vi "rawpower2totalprad.vi"(3 "PowerArray [W]":sgl[][](array[numeric]), 4 "No. of Samples\n[TOA / Sample Rate]":u32=10000, 5 "kbolott_and_volume":dbl[][](array[numeric])) -> (0 "full P_rad [MW] HBC":dbl[](array[numeric]), 1 "full P_rad [MW] VBC":dbl[](array[numeric]), 2 "corrected PowerArray":dbl[][](array[numeric]))   [LabVIEW 2014]
panel:
  out "sample2":i32
  out "sample":i32
  out "channel VBC":i32
  out "V_Cam 2":dbl format="%#_13g"
  out "channelListVBC":i32[](array[numeric])
  out "sample array [MW] 2":dbl[](array[numeric])
  out "constant 2":dbl
  out "element 2":sgl
  out "volume/kbolott 2":dbl
  out "element after 2":dbl
  out "kbolott 2":dbl
  out "volume 2":dbl
  out "constant*geom 2":dbl
  out "test plot":cluster{cluster{i32, "element":dbl}[]}[](graph)
  out "Nsample array":i32[](array[numeric])
  out "channel subarray":sgl[](array[numeric])
  out "offset channel":sgl
  out "channel":i32
  out "power size":i32[](array[numeric])
  out "offset size":i32[](array[numeric])
  out "power offset all 128":dbl[](array[numeric])
  out "start subarray":sgl[][](array[numeric])
  in  "channel\noffset":i32
  out "constant*geom":dbl
  out "volume":dbl
  out "kbolott":dbl
  out "element after":dbl
  out "volume/kbolott":dbl
  out "element":sgl
  in  "Nchannels":i32=32
  out "sample array [MW]":dbl[](array[numeric])
  out "constant":dbl
  out "V_Cam":dbl format="%#_13g"
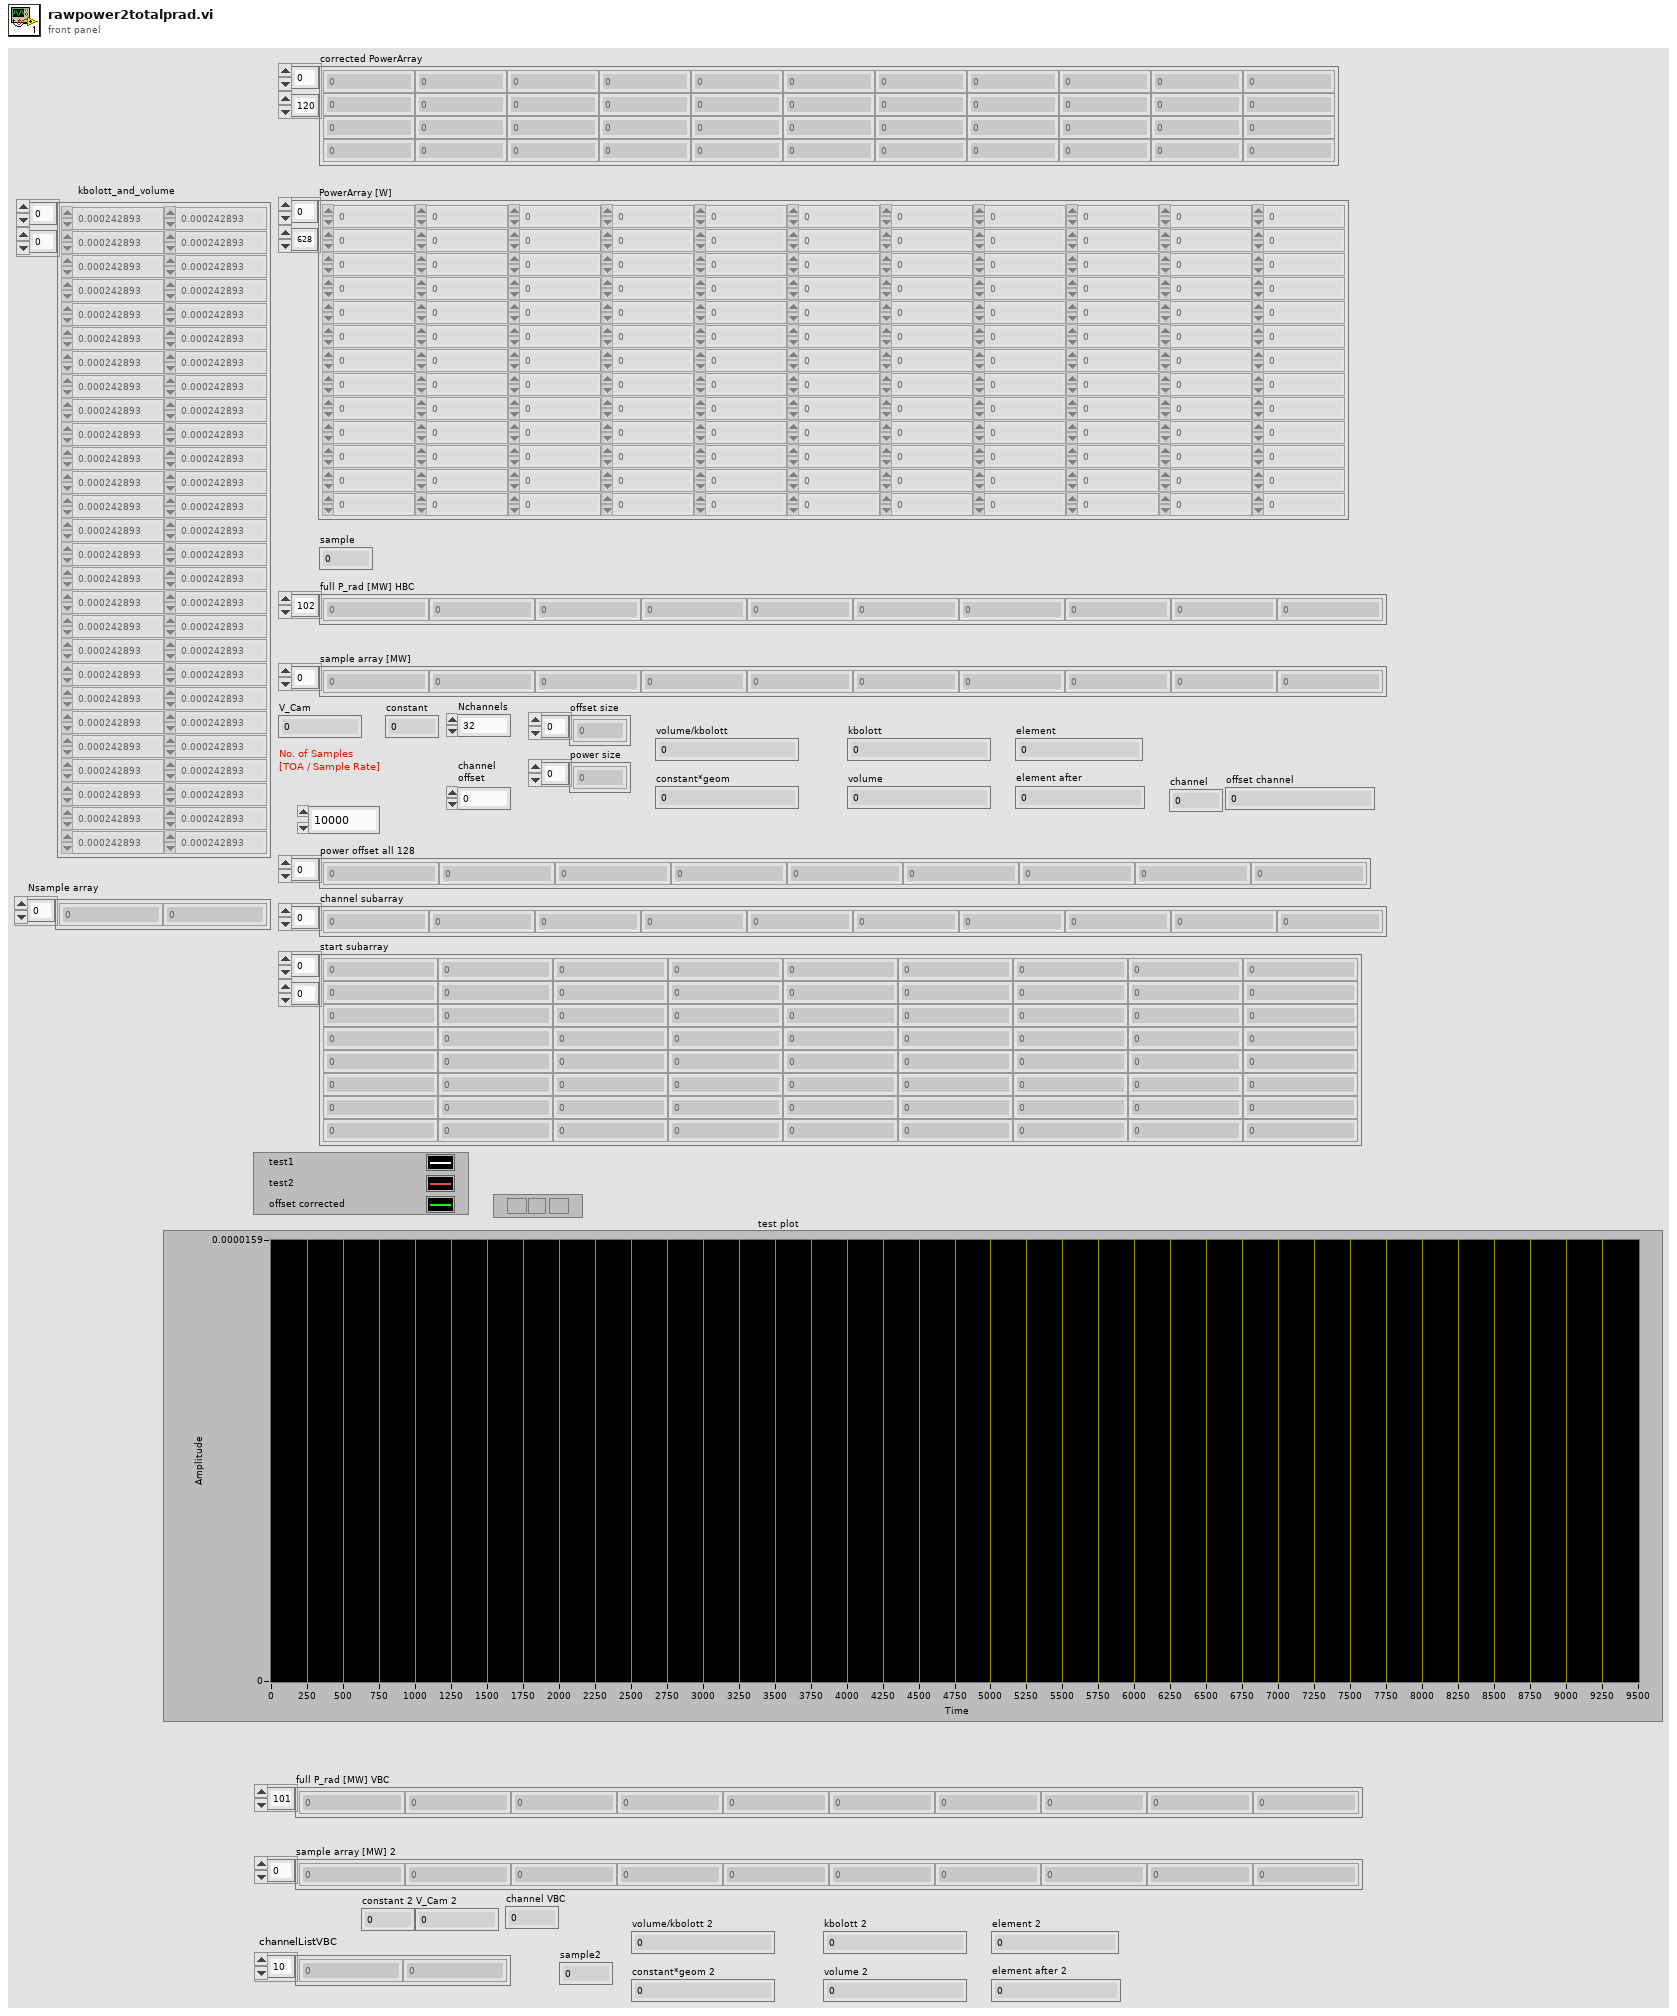
[diagram p1: front panel]
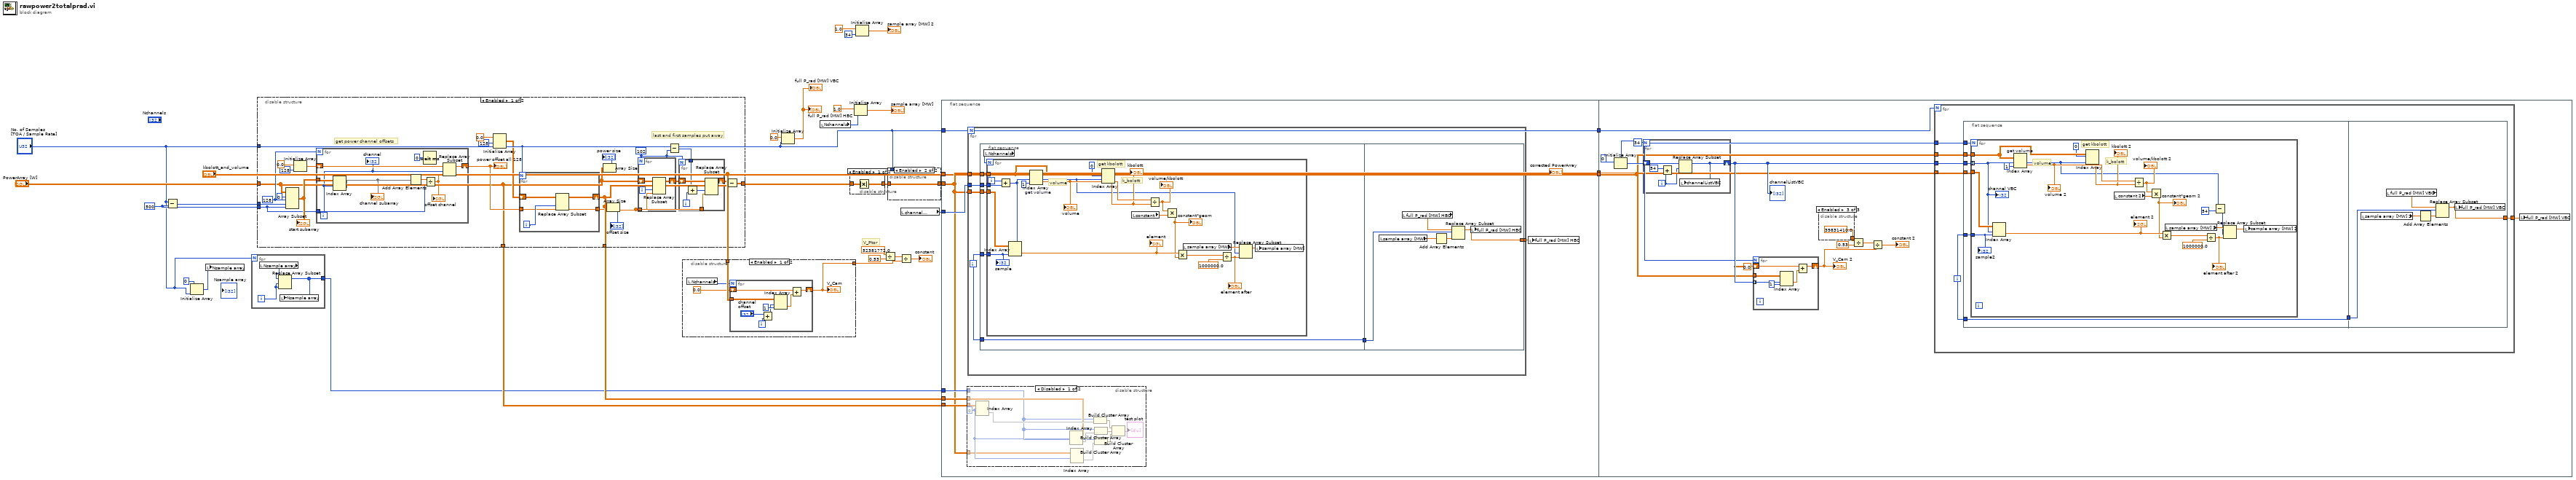
[diagram p0: block diagram]
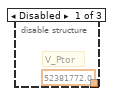
[diagram p3: hidden frame]
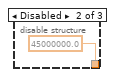
[diagram p4: hidden frame]
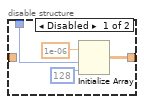
[diagram p7: hidden frame]
diagram:
  w14 = u32 500 ("y")
  # "V_Ptor"
  n1 = Subtract(x="No. of Samples\n[TOA / Sample Rate]", y=w14) -> (x-y=w15:u32)
  n2 = Initialize Array(0, "No. of Samples\n[TOA / Sample Rate]") -> (w19:i32[])
  n3 = local write "Nsample array"(w19) -> ()
  n4 = for {
    N: "No. of Samples\n[TOA / Sample Rate]" -> [_]
    tunnel: [w31] -> w16
    i -> [w32]
    n5 = local read "Nsample array"() -> (w33:i32[])
    n6 = Replace Array Subset(array=w33, new element=w32, index=w32) -> (w31:i32[])
    n7 = local write "Nsample array"(w31) -> ()
  }
  n8 = disable-structure shown="Enabled" {
    disable-tunnel: "PowerArray [W]" -> [w40 w80]
    disable-tunnel: [w43 w80] -> w12
    disable-tunnel: "No. of Samples\n[TOA / Sample Rate]" -> [w36 _]
    disable-tunnel: [w40 _] -> w18
    disable-tunnel: [w44 _] -> w17
    disable-tunnel: w15 -> [w42 _]
    disable-tunnel: w14 -> [w41 _]
    frame Enabled {
      w35 = 102
      w45 = 128 ("length")
      # "last and first samples put away"
      # "get power channel offsets"
      n9 = Array Subset(array=w40, index (row)=0 ("index"), length (row)=w45, index (col)=w42, length (col)=w41) -> (w53:sgl[][])
      "start subarray" <- w53
      n10 = Initialize Array(0.0 ("element"), 128 ("dimension size")) -> (w52:dbl[])
      n11 = for {
        N: w45 -> [_]
        tunnel: w53 -> [w73]
        tunnel: w41 -> [w75]
        shift-right: [w76] -> w49
        shift-left: w52 -> [w78]
        i -> [w72]
        n12 = Index Array(array=w73, index (row)=w72) -> (element=w71:sgl[])  [unwired: 1 in]
        "channel subarray" <- w71
        n13 = Add Array Elements(numeric array=w71) -> (sum=w79:sgl)
        n14 = Wait (ms)(milliseconds to wait=u32 0) -> ()  [unwired: 1 out]
        n15 = Divide(x=w79, y=w75) -> (x/y=w77:sgl)
        "offset channel" <- w77
        n16 = Replace Array Subset(array=w78, new element=w77, index=w72) -> (w76:dbl[])
        "channel" <- w72
      }
      "power offset all 128" <- w49
      n17 = Initialize Array(0.0 ("element"), 128 ("dimension size"), w36) -> (w50:dbl[][])
      n18 = for {
        N: w36 -> [_]
        shift-right: [w68] -> w44
        shift-left: w50 -> [w70]
        tunnel: w49 -> [w67]
        tunnel: [w67] -> w37
        i -> [w69]
        n19 = Replace Array Subset(array=w70, new element=w67, index (col)=w69) -> (w68:dbl[][])  [unwired: 1 in]
      }
      n20 = Array Size(array=w40) -> (size(s)=→"power size":i32[])
      n21 = Array Size(array=w44) -> (size(s)=→"offset size":i32[])
      n22 = for {
        N: w35 -> [_]
        shift-right: [w65] -> w39
        shift-left: w40 -> [w66]
        tunnel: w37 -> [w63]
        i -> [w64]
        n23 = Replace Array Subset(array=w66, new element=w63, index (col)=w64) -> (w65:sgl[][])  [unwired: 1 in]
      }
      n24 = Subtract(x=w36, y=w35) -> (x-y=w34:u32)
      n25 = for {
        N: w35 -> [_]
        shift-right: [w61] -> w38
        shift-left: w39 -> [w62]
        tunnel: w37 -> [w60]
        tunnel: w34 -> [w59]
        i -> [w58]
        n26 = Add(x=w59, y=w58) -> (x+y=w57:u32)
        n27 = Replace Array Subset(array=w62, new element=w60, index (col)=w57) -> (w61:sgl[][])  [unwired: 1 in]
      }
      n28 = Subtract(x=w38, y=w44) -> (x-y=w43:dbl[][])
    }
    frame Disabled {
    }
  }
  n29 = disable-structure shown="Enabled" {
    disable-tunnel: "kbolott_and_volume" -> [w84 _]
    disable-tunnel: [w81 _] -> w22
    frame Enabled {
      n30 = local read "Nchannels"() -> (w83:i32)
      n31 = for {
        N: w83 -> [_]
        tunnel: w84 -> [w92]
        shift-right: [w88] -> w81
        shift-left: 0.0 ("V_Cam") -> [w89]
        i -> [w86]
        n32 = Add(x="channel\noffset", y=w86) -> (x+y=w87:i32)
        n33 = Index Array(array=w92, index (row)=w87, index (col)=1 ("disabled index (col)")) -> (element=w91:dbl)
        n34 = Add(x=w89, y=w91) -> (x+y=w88:dbl)
      }
      "V_Cam" <- w81
    }
    frame Disabled {
    }
  }
  n35 = Initialize Array(0.0 ("element"), "No. of Samples\n[TOA / Sample Rate]") -> (→"full P_rad [MW] HBC" →"full P_rad [MW] VBC":dbl[])
  n36 = local read "Nchannels"() -> (w27:i32)
  n37 = disable-structure shown="Enabled" {
    disable-tunnel: [w94 w95] -> w21
    disable-tunnel: w12 -> [w93 w95]
    frame Enabled {
      n38 = Absolute Value(x=w93) -> (abs(x)=w94:dbl[][])
    }
    frame Disabled {
    }
  }
  n39 = Initialize Array(1.0 ("element"), w27) -> (→"sample array [MW]":dbl[])
  n40 = Initialize Array(1.0 ("element"), 34 ("dimension size")) -> (→"sample array [MW] 2":dbl[])
  n41 = Divide(x=52381772.0, y=0.53) -> (x/y=w25:dbl)
  n42 = disable-structure shown="Enabled" {
    disable-tunnel: "No. of Samples\n[TOA / Sample Rate]" -> [w98 _]
    disable-tunnel: [w96 w100] -> w9
    disable-tunnel: w21 -> [_ w100]
    frame Disabled {
      n43 = Initialize Array(1e-06 ("element"), w98, 128 ("dimension size")) -> (w96:dbl[][])
    }
    frame Enabled {
    }
  }
  n44 = Divide(x=w25, y=w22) -> (x/y=→"constant":dbl)
  n45 = local read "channel\noffset"() -> (w23:i32)
  n46 = flat-sequence {
    tunnel: w23 -> [w108]
    tunnel: w18 -> [w106]
    tunnel: w17 -> [w105]
    tunnel: w16 -> [w104]
    tunnel: w9 -> [w102]
    tunnel: [w103] -> w8
    tunnel: "No. of Samples\n[TOA / Sample Rate]" -> [w103]
    tunnel: [w102] -> w6
    tunnel: [w101] -> w5
    tunnel: "kbolott_and_volume" -> [w101]
    tunnel: w8 -> [w159]
    tunnel: w6 -> [w157]
    tunnel: w5 -> [w158]
    frame #0 {
      n47 = disable-structure shown="Disabled" {
        disable-tunnel: w106 -> [w117 _]
        disable-tunnel: w105 -> [w115 _]
        disable-tunnel: w104 -> [w112 _]
        disable-tunnel: w102 -> [w109 _]
        frame Disabled {
          w111 = 0 ("index (row)")
          n48 = Index Array(array=w117, index (row)=w111) -> (element=w116:sgl[])  [unwired: 1 in]
          n49 = Index Array(array=w115, index (row)=w111) -> (element=w114:dbl[])  [unwired: 1 in]
          n50 = Index Array(array=w109, index (row)=w111) -> (element=w110:dbl[])  [unwired: 1 in]
          n51 = Build Cluster Array(w112, w116) -> (w118:cluster{i32, sgl}[])
          n52 = Build Cluster Array(w112, w114) -> (w120:cluster{i32, "element":dbl}[])
          n53 = Build Cluster Array(w112, w110) -> (w113:cluster{i32, dbl}[])
          n54 = Build Cluster Array(w118, w120, w113) -> (→"test plot":cluster{cluster{i32, "element":dbl}[]}[])
        }
        frame Enabled {
        }
      }
      n55 = for {
        N: w103 -> [_]
        tunnel: w102 -> [w126]
        tunnel: w101 -> [w125]
        tunnel: w108 -> [w122]
        tunnel: [w121] -> w107
        i -> [w123]
        n56 = flat-sequence {
          tunnel: w126 -> [w131]
          tunnel: w125 -> [w130]
          tunnel: w123 -> [w129]
          tunnel: [w128] -> w124
          tunnel: w123 -> [w128]
          tunnel: w122 -> [w127]
          tunnel: w124 -> [w155]
          tunnel: [w152] -> w121
          frame #0 {
            n57 = local read "Nchannels"() -> (w132:i32)
            n58 = for {
              N: w132 -> [_]
              tunnel: w131 -> [w148]
              tunnel: w130 -> [w150]
              tunnel: w129 -> [w147]
              tunnel: w127 -> [w133]
              i -> [w135]
              # "get kbolott"
              # "k_bolott"
              # "volume"
              n59 = Add(x=w135, y=w133) -> (x+y=w134:i32)
              n60 = Index Array(array=w148, index (row)=w134, index (col)=w147) -> (element=w144:dbl)
              "element" <- w144
              n61 = Index Array "get volume"(array=w150, index (row)=w134, index (col)=1 ("disabled index (col)")) -> (element=w142:dbl)
              "volume" <- w142
              n62 = Index Array(array=w150, index (row)=w134, index (col)=0 ("disabled index (col)")) -> (element=w136:dbl)
              "kbolott" <- w136
              n63 = local read "constant"() -> (w139:dbl)
              n64 = Divide(x=w142, y=w136) -> (x/y=w141:dbl)
              "volume/kbolott" <- w141
              n65 = Multiply(x=w141, y=w139) -> (x*y=w140:dbl)
              "constant*geom" <- w140
              n66 = Multiply(x=w144, y=w140) -> (x*y=w143:dbl)
              n67 = local read "sample array [MW]"() -> (w138:dbl[])
              n68 = Divide(x=w143, y=1000000.0) -> (x/y=w145:dbl)
              "element after" <- w145
              n69 = Replace Array Subset(array=w138, new element=w145, index=w134) -> (w137:dbl[])
              n70 = local write "sample array [MW]"(w137) -> ()
              "sample" <- w147
            }
          }
          frame #1 {
            n71 = local read "sample array [MW]"() -> (w153:dbl[])
            n72 = local read "full P_rad [MW] HBC"() -> (w156:dbl[])
            n73 = Add Array Elements(numeric array=w153) -> (sum=w154:dbl)
            n74 = Replace Array Subset(array=w156, new element=w154, index=w155) -> (w152:dbl[])
            n75 = local write "full P_rad [MW] HBC"(w152) -> ()
          }
        }
      }
      n76 = local write "full P_rad [MW] HBC"(w107) -> ()
      "corrected PowerArray" <- w102
    }
    frame #1 {
      w168 = 34
      n77 = Initialize Array(0, w168) -> (w169:i32[])
      n78 = for {
        N: w168 -> [_]
        shift-right: [w180] -> w170
        shift-left: w169 -> [w181]
        i -> [w184]
        n79 = Add(x=54, y=w184) -> (x+y=w182:i32)
        n80 = Replace Array Subset(array=w181, new element=w182, index=w184) -> (w180:i32[])
        n81 = local write "channelListVBC"(w180) -> ()
      }
      "channelListVBC" <- w170
      n82 = for {
        N: w168 -> [_]
        tunnel: w158 -> [w179]
        shift-right: [w175] -> w165
        shift-left: 0.0 ("V_Cam") -> [w176]
        tunnel: w170 -> [w174] mode=indexing
        n83 = Index Array(array=w179, index (row)=w174, index (col)=1 ("disabled index (col)")) -> (element=w178:dbl)
        n84 = Add(x=w176, y=w178) -> (x+y=w175:dbl)
      }
      "V_Cam 2" <- w165
      n85 = disable-structure shown="Enabled" {
        disable-tunnel: [52381772.0 45000000.0 39831410.0] -> w160
        frame Disabled {
          # "V_Ptor"
        }
        frame Disabled {
        }
        frame Enabled {
        }
      }
      n86 = Divide(x=w160, y=0.53) -> (x/y=w162:dbl)
      n87 = Divide(x=w162, y=w165) -> (x/y=→"constant 2":dbl)
      n88 = for {
        N: w159 -> [_]
        tunnel: w157 -> [w191]
        tunnel: w158 -> [w190]
        tunnel: [w187] -> w166
        tunnel: w168 -> [w186]
        tunnel: w170 -> [w185]
        i -> [w188]
        n89 = flat-sequence {
          tunnel: w191 -> [w197]
          tunnel: w190 -> [w196]
          tunnel: w188 -> [w195]
          tunnel: [w194] -> w189
          tunnel: w188 -> [w194]
          tunnel: w186 -> [w193]
          tunnel: w185 -> [w192]
          tunnel: w189 -> [w220]
          tunnel: [w217] -> w187
          frame #0 {
            n90 = for {
              N: w193 -> [_]
              tunnel: w197 -> [w213]
              tunnel: w196 -> [w215]
              tunnel: w195 -> [w200]
              tunnel: w192 -> [w201] mode=indexing
              # "get kbolott"
              # "k_bolott"
              # "volume"
              n91 = Index Array(array=w213, index (row)=w201, index (col)=w200) -> (element=w210:dbl)
              "element 2" <- w210
              n92 = Index Array "get volume"(array=w215, index (row)=w201, index (col)=1 ("disabled index (col)")) -> (element=w208:dbl)
              "volume 2" <- w208
              n93 = Index Array(array=w215, index (row)=w201, index (col)=0 ("disabled index (col)")) -> (element=w202:dbl)
              "kbolott 2" <- w202
              n94 = local read "constant 2"() -> (w205:dbl)
              n95 = Divide(x=w208, y=w202) -> (x/y=w207:dbl)
              "volume/kbolott 2" <- w207
              n96 = Multiply(x=w207, y=w205) -> (x*y=w206:dbl)
              "constant*geom 2" <- w206
              n97 = Multiply(x=w210, y=w206) -> (x*y=w209:dbl)
              n98 = local read "sample array [MW] 2"() -> (w204:dbl[])
              n99 = Divide(x=w209, y=1000000.0) -> (x/y=w211:dbl)
              "element after 2" <- w211
              n100 = Subtract(x=w201, y=54) -> (x-y=w199:i32)
              n101 = Replace Array Subset(array=w204, new element=w211, index=w199) -> (w203:dbl[])
              n102 = local write "sample array [MW] 2"(w203) -> ()
              "channel VBC" <- w201
              "sample2" <- w200
            }
          }
          frame #1 {
            n103 = local read "sample array [MW] 2"() -> (w218:dbl[])
            n104 = local read "full P_rad [MW] VBC"() -> (w221:dbl[])
            n105 = Add Array Elements(numeric array=w218) -> (sum=w219:dbl)
            n106 = Replace Array Subset(array=w221, new element=w219, index=w220) -> (w217:dbl[])
            n107 = local write "full P_rad [MW] VBC"(w217) -> ()
          }
        }
      }
      n108 = local write "full P_rad [MW] VBC"(w166) -> ()
    }
  }
